vi "Util.Pic.GIF.Write.vi"(5 "overwrite? (false)":bool, 6 "error in (no error)":errorcluster, 7 "Delay (ms)":u32, 8 "images data":T1[](array[typedef]), 9 "path to GIF file":path) -> (0 "error out":errorcluster)   [LabVIEW 2014]
doc: "Writes a multi-frame (animated) Compuserve GIF file. If no path is specified, a file dialog is used to find the file."
uses:
  Util.Pic.t.image.ctl
panel:
  # "Util.Pic.GIF.Write.vi\n\nWrites a multi-frame (animated) Compuserve GIF file. If no path is specified, a file dialog is used to find the file.\n\nNOTICE -- YOU MUST LEAVE THIS NOTICE IN PLACE.  PER THE TERMS OF THE LICENSE BELOW, YOU MAY SUBLICENSE THIS SOFTWARE \nIN ANY WAY THAT DOES NOT CONFLICT WITH THIS LICENSE.\n\n### BSD License (http://www.opensource.org/licenses/bsd-license.php) Begin ###\n \nCopyright (c) 2007, Bill Clench <bclench@yahoo.com>\n\nAll rights reserved.\n\nRedistribution and use in source and binary forms, with or without modification, are permitted provided that the following conditions are met:\n\n    * Redistributions of source code must retain the above copyright notice, this list of conditions and the following disclaimer.\n    * Redistributions in binary form must reproduce the above copyright notice, this list of conditions and the following disclaimer in the \n       documentation and/or other materials provided with the distribution.\n\nTHIS SOFTWARE IS PROVIDED BY THE COPYRIGHT HOLDERS AND CONTRIBUTORS \"AS IS\" AND ANY EXPRESS OR IMPLIED WARRANTIES, \nINCLUDING, BUT NOT LIMITED TO, THE IMPLIED WARRANTIES OF MERCHANTABILITY AND FITNESS FOR A PARTICULAR PURPOSE ARE \nDISCLAIMED. IN NO EVENT SHALL THE COPYRIGHT OWNER OR CONTRIBUTORS BE LIABLE FOR ANY DIRECT, INDIRECT, INCIDENTAL,\n SPECIAL, EXEMPLARY, OR CONSEQUENTIAL DAMAGES (INCLUDING, BUT NOT LIMITED TO, PROCUREMENT OF SUBSTITUTE GOODS OR \nSERVICES; LOSS OF USE, DATA, OR PROFITS; OR BUSINESS INTERRUPTION) HOWEVER CAUSED AND ON ANY THEORY OF LIABILITY, \nWHETHER IN CONTRACT, STRICT LIABILITY, OR TORT (INCLUDING NEGLIGENCE OR OTHERWISE) ARISING IN ANY WAY OUT OF THE USE \nOF THIS SOFTWARE, EVEN IF ADVISED OF THE POSSIBILITY OF SUCH DAMAGE.\n\n### BSD License End ###"
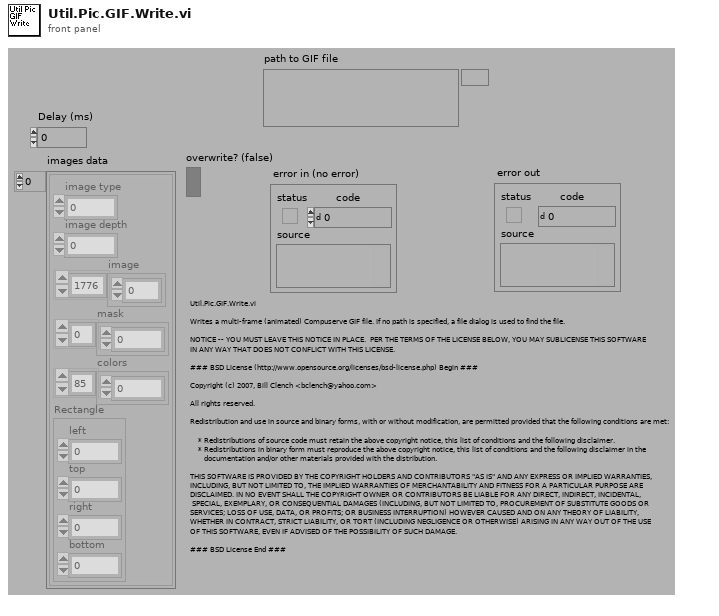
[diagram p1: front panel]
types:
  T1 = typedef "Util.Pic.t.image.ctl" = cluster{"image type":i32, "image depth":i32, "image":u8[], "mask":u8[], "colors":u32[], "Rectangle":cluster{"left":i16, "top":i16, "right":i16, "bottom":i16}}
  T2 = enum16{"open", "replace", "create", "open or create", "replace or create", "replace or create with confirmation"}
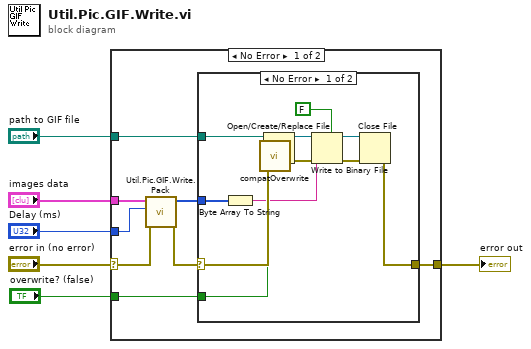
[diagram p0: block diagram]
diagram:
  n1 = case shown="No Error" "error in (no error)" {
    selector: "error in (no error)" -> [w11 w28]
    tunnel: "images data" -> [w14 _]
    tunnel: [w13 w28] -> w5
    tunnel: "path to GIF file" -> [w10 _]
    tunnel: "overwrite? (false)" -> [w12 _]
    tunnel: "Delay (ms)" -> [w7 _]
    frame No Error {
      n2 = call "Util.Pic.GIF.Write.Pack.vi"("error in (no error)"=w11, "Delay (ms)"=w7, "Images"=w14) -> ("error out"=w9:errorcluster, "Array"=w8:u8[])  [unwired: 7 in]
      n3 = case shown="No Error" w9 {
        selector: w9 -> [w26 w27]
        tunnel: [w25 w27] -> w13
        tunnel: w8 -> [w24 _]
        tunnel: w10 -> [w17 _]
        tunnel: w12 -> [w22 _]
        frame No Error {
          n4 = Byte Array To String(unsigned byte array=w24) -> (string=w23:string)
          n5 = call <vilib>:"compatOverwrite.vi"("overwrite (F)"=w22) -> ("overwrite?"=w15:T2)
          n6 = Open/Create/Replace File(file path (use dialog)=w17, error in=w26, operation (0:open)=w15) -> (refnum out=w21:refnum<file>, error out=w20:errorcluster)  [unwired: 3 in, 1 out]
          n7 = Write to Binary File(file (use dialog)=w21, data=w23, error in=w20, 5:FALSE ("prepend array or string size? (T)")) -> (refnum out=w19:refnum<file>, error out=w18:errorcluster)  [unwired: 2 in, 1 out]
          n8 = Close File(refnum=w19, error in=w18) -> (error out=w25:errorcluster)  [unwired: 1 out]
        }
        frame Error {
        }
      }
    }
    frame Error {
    }
  }
  "error out" <- w5
